vi "Write-Value.vi"(0 "Quick-GUI-Update in":refnum<class "Quick-GUI-Update.lvclass">, 2 "Label":string, 7 "Value In":variant, 11 "error in (no error)":errorcluster) -> (4 "Quick-GUI-Update out":refnum<class "Quick-GUI-Update.lvclass">, 8 "Status":u8[](array[numeric]), 15 "error out":errorcluster)   [LabVIEW 2020, in "Easy GUI Operation.lvlib" / "Quick-GUI-Update.lvclass"]
doc: "<b>Status</b>\n0 ---> Value Not Updated.\n1 ---> Value Updated using <b>\"Set Ctrl Value By Index\"</b> function.\n2 ---> Value Updated using <b>\"Value\"</b> Property."
uses:
  Quick-GUI-Update.lvclass
  Quick-GUI-Update.lvclass/Quick-GUI-Update.ctl
  <vilib>/Utility/Data Type/NI_Data Type.lvlib
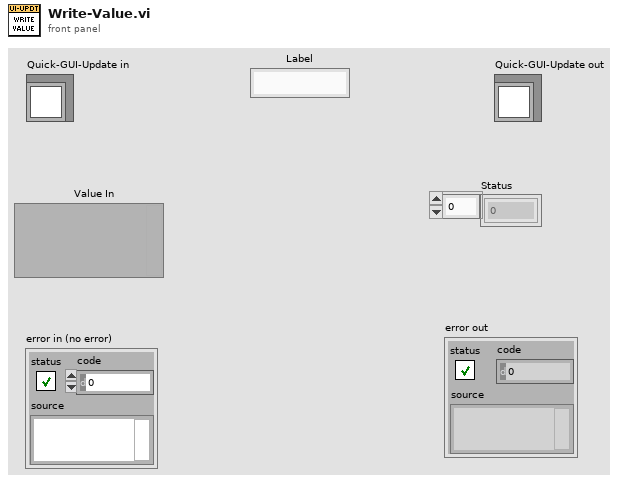
[diagram p1: front panel]
types:
  T1 = map{string, set{cluster{"Ctrl-Ref":refnum<vi>, "Ctrl Index":i32, "Class-Name":string, "Class ID":u32}}}
  T2 = set{cluster{"Ctrl-Ref":refnum<vi>, "Ctrl Index":i32, "Class-Name":string, "Class ID":u32}}
  T3 = typedef "NI_Data Type.lvlib/Data Type.ctl" = enum8{"Invalid Type", "Void", "I8", "I16", "I32", "I64", "U8", "U16", "U32", "U64", "Single Float", "Double Float", "Extended Float", "Single Complex", "Double Complex", "Extended Complex", "Enum U8", "Enum U16", "Enum U32", "Enum U64", "Single Float With Unit", "Double Float With Unit", "Extended Float With Unit", "Single Complex with Unit", "Double Complex with Unit", "Extended Complex with Unit", "Boolean", "String", "Path", "Picture", "Tag", "Array", "Cluster", "Variant", "LV Variant", "Waveform", "Timestamp", "Digital Waveform", "Digital Data", "ExpressData", "Refnum", "External Data", "VI", "Poly VI", "LabVIEW Class Instance", "Fixed Point", "Set Collection", "Map Collection"}
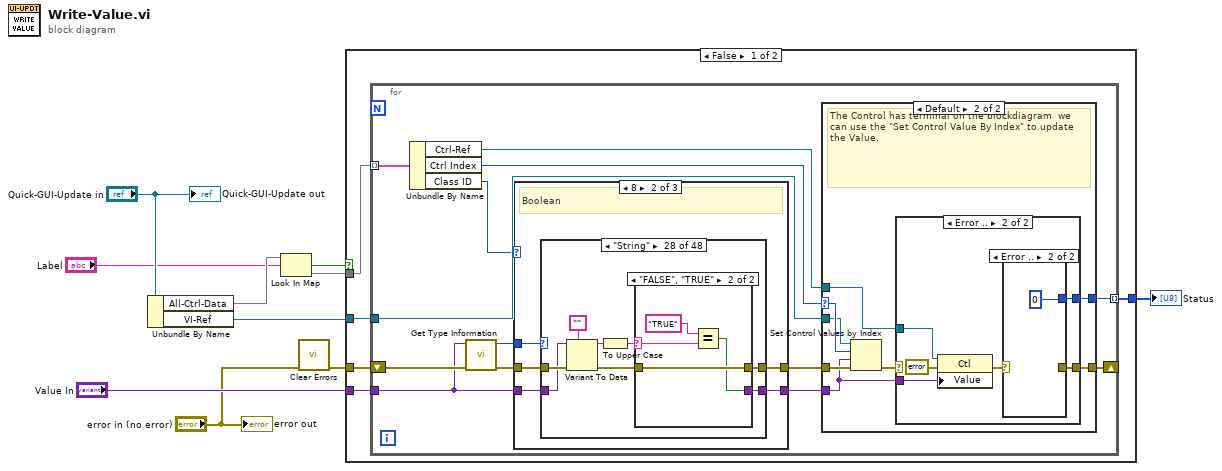
[diagram p0: block diagram]
diagram:
  n1 = Unbundle By Name("Quick-GUI-Update in") -> ("All-Ctrl-Data"=w8:T1, "VI-Ref"=w4:refnum<vi>)
  n2 = Look In Map(map=w8, key="Label") -> (key not found?=w6:bool, value=w5:T2)  [unwired: 1 in]
  n3 = call <vilib>:"Clear Errors.vi"("error in (no error)"="error in (no error)") -> ("error out"=w2:errorcluster)  [unwired: 5 in, 1 out]
  n4 = case shown="False" w6 {
    tunnel: w2 -> [w13 _]
    tunnel: "Value In" -> [w14 _]
    tunnel: w5 -> [w11 _]
    tunnel: w4 -> [w15 _]
    tunnel: [w12 _] -> w3
    frame False {
      n5 = for {
        tunnel: w11 -> [w26] mode=indexing
        tunnel: w15 -> [w24]
        tunnel: w14 -> [w19]
        shift-right: [w25] -> _
        shift-left: w13 -> [w22]
        tunnel: [w23] -> w12 mode=indexing
        n6 = Unbundle By Name(w26) -> ("Ctrl-Ref"=w27:refnum<vi>, "Ctrl Index"=w28:i32, "Class ID"=w21:u32)
        n7 = call <vilib>:"Get Type Information.vi"("error in (no error)"=w22, "variant"=w19) -> ("error out"=w18:errorcluster, "type"=w20:T3)  [unwired: 5 in, 3 out]
        n8 = case shown="8" w21 {
          tunnel: w20 -> [_ w35 w149]
          tunnel: w19 -> [w29 w32 w146]
          tunnel: w18 -> [w30 w34 w148]
          tunnel: [w30 w33 w147] -> w17
          tunnel: [w29 w31 w145] -> w16
          frame Default {
          }
          frame 8 {
            # "Boolean"
            n9 = case shown="\"String\"" w35 {
              tunnel: w34 -> [w37 w39 w41 w43 w45 w47 w49 w51 w53 w55 w57 w59 w61 w63 w65 w67 w69 w71 w73 w75 w77 w79 w81 w83 w85 w87 w89 w97 w106 w108 w110 w112 w114 w116 w118 w120 w122 w124 w126 w128 w130 w132 w134 w136 w138 w140 w142 w144]
              tunnel: [w37 w39 w41 w43 w45 w47 w49 w51 w53 w55 w57 w59 w61 w63 w65 w67 w69 w71 w73 w75 w77 w79 w81 w83 w85 w87 w89 w91 w106 w108 w110 w112 w114 w116 w118 w120 w122 w124 w126 w128 w130 w132 w134 w136 w138 w140 w142 w144] -> w33
              tunnel: w32 -> [w36 w38 w40 w42 w44 w46 w48 w50 w52 w54 w56 w58 w60 w62 w64 w66 w68 w70 w72 w74 w76 w78 w80 w82 w84 w86 w88 w96 w105 w107 w109 w111 w113 w115 w117 w119 w121 w123 w125 w127 w129 w131 w133 w135 w137 w139 w141 w143]
              tunnel: [w36 w38 w40 w42 w44 w46 w48 w50 w52 w54 w56 w58 w60 w62 w64 w66 w68 w70 w72 w74 w76 w78 w80 w82 w84 w86 w88 w92 w105 w107 w109 w111 w113 w115 w117 w119 w121 w123 w125 w127 w129 w131 w133 w135 w137 w139 w141 w143] -> w31
              frame "Invalid Type" {
              }
              frame "Void" {
              }
              frame "I8" {
              }
              frame "I16" {
              }
              frame "I32" {
              }
              frame "I64" {
              }
              frame "U8" {
              }
              frame "U16" {
              }
              frame "U32" {
              }
              frame "U64" {
              }
              frame "Single Float" {
              }
              frame "Double Float" {
              }
              frame "Extended Float" {
              }
              frame "Single Complex" {
              }
              frame "Double Complex" {
              }
              frame "Extended Complex" {
              }
              frame "Enum U8" {
              }
              frame "Enum U16" {
              }
              frame "Enum U32" {
              }
              frame "Enum U64" {
              }
              frame "Single Float With Unit" {
              }
              frame "Double Float With Unit" {
              }
              frame "Extended Float With Unit" {
              }
              frame "Single Complex with Unit" {
              }
              frame "Double Complex with Unit" {
              }
              frame "Extended Complex with Unit" {
              }
              frame "Boolean" {
              }
              frame "String" {
                n10 = Variant To Data(error in=w97, type="" ("Empty String Constant"), Variant=w96) -> (data=w95:string, error out=w93:errorcluster)
                n11 = To Upper Case(1:w95) -> (0:w94:string)
                n12 = case shown="\"FALSE\", \"TRUE\"" w94 {
                  selector: w94 -> [w99 w103]
                  tunnel: w93 -> [w100 w104]
                  tunnel: [w98 w101] -> w92
                  tunnel: [w100 w104] -> w91
                  frame Default {
                    n13 = To Variant(anything=w99) -> (Variant=w98:variant)
                  }
                  frame "FALSE", "TRUE" {
                    n14 = Equal?(x="TRUE", y=w103) -> (x = y?=w101:bool)
                  }
                }
              }
              frame "Path" {
              }
              frame "Picture" {
              }
              frame "Tag" {
              }
              frame "Array" {
              }
              frame "Cluster" {
              }
              frame "Variant" {
              }
              frame "LV Variant" {
              }
              frame "Waveform" {
              }
              frame "Timestamp" {
              }
              frame "Digital Waveform" {
              }
              frame "Digital Data" {
              }
              frame "ExpressData" {
              }
              frame "Refnum" {
              }
              frame "External Data" {
              }
              frame "VI" {
              }
              frame "Poly VI" {
              }
              frame "LabVIEW Class Instance" {
              }
              frame "Fixed Point" {
              }
              frame "Set Collection" {
              }
              frame "Map Collection" {
              }
            }
          }
          frame 27 {
            # "String"
            n15 = case shown="\"Invalid Type\"" w149 {
              tunnel: w148 -> [w151 w153 w155 w157 w159 w161 w163 w165 w167 w169 w171 w173 w175 w177 w179 w181 w183 w185 w187 w189 w191 w193 w195 w197 w199 w201 w208 w210 w212 w214 w216 w218 w220 w222 w224 w226 w228 w230 w232 w234 w236 w238 w240 w242 w244 w246 w248 w250]
              tunnel: [w151 w153 w155 w157 w159 w161 w163 w165 w167 w169 w171 w173 w175 w177 w179 w181 w183 w185 w187 w189 w191 w193 w195 w197 w199 w201 w206 w210 w212 w214 w216 w218 w220 w222 w224 w226 w228 w230 w232 w234 w236 w238 w240 w242 w244 w246 w248 w250] -> w147
              tunnel: w146 -> [w150 w152 w154 w156 w158 w160 w162 w164 w166 w168 w170 w172 w174 w176 w178 w180 w182 w184 w186 w188 w190 w192 w194 w196 w198 w200 w205 w209 w211 w213 w215 w217 w219 w221 w223 w225 w227 w229 w231 w233 w235 w237 w239 w241 w243 w245 w247 w249]
              tunnel: [w150 w152 w154 w156 w158 w160 w162 w164 w166 w168 w170 w172 w174 w176 w178 w180 w182 w184 w186 w188 w190 w192 w194 w196 w198 w200 w202 w209 w211 w213 w215 w217 w219 w221 w223 w225 w227 w229 w231 w233 w235 w237 w239 w241 w243 w245 w247 w249] -> w145
              frame "Invalid Type" {
              }
              frame "Void" {
              }
              frame "I8" {
              }
              frame "I16" {
              }
              frame "I32" {
              }
              frame "I64" {
              }
              frame "U8" {
              }
              frame "U16" {
              }
              frame "U32" {
              }
              frame "U64" {
              }
              frame "Single Float" {
              }
              frame "Double Float" {
              }
              frame "Extended Float" {
              }
              frame "Single Complex" {
              }
              frame "Double Complex" {
              }
              frame "Extended Complex" {
              }
              frame "Enum U8" {
              }
              frame "Enum U16" {
              }
              frame "Enum U32" {
              }
              frame "Enum U64" {
              }
              frame "Single Float With Unit" {
              }
              frame "Double Float With Unit" {
              }
              frame "Extended Float With Unit" {
              }
              frame "Single Complex with Unit" {
              }
              frame "Double Complex with Unit" {
              }
              frame "Extended Complex with Unit" {
              }
              frame "Boolean" {
                n16 = Variant To Data(error in=w208, type=FALSE, Variant=w205) -> (data=w203:bool, error out=w207:errorcluster)
                n17 = Format Into String(error in=w207, w203) -> (resulting string=w202:string, error out=w206:errorcluster)  [unwired: 2 in]
              }
              frame "String" {
              }
              frame "Path" {
              }
              frame "Picture" {
              }
              frame "Tag" {
              }
              frame "Array" {
              }
              frame "Cluster" {
              }
              frame "Variant" {
              }
              frame "LV Variant" {
              }
              frame "Waveform" {
              }
              frame "Timestamp" {
              }
              frame "Digital Waveform" {
              }
              frame "Digital Data" {
              }
              frame "ExpressData" {
              }
              frame "Refnum" {
              }
              frame "External Data" {
              }
              frame "VI" {
              }
              frame "Poly VI" {
              }
              frame "LabVIEW Class Instance" {
              }
              frame "Fixed Point" {
              }
              frame "Set Collection" {
              }
              frame "Map Collection" {
              }
            }
          }
        }
        n18 = case shown="Default" w28 {
          selector: w28 -> [_ w267]
          tunnel: w27 -> [w256 w265]
          tunnel: w16 -> [w255 w262]
          tunnel: w17 -> [w254 w264]
          tunnel: [w251 w263] -> w25
          tunnel: w24 -> [_ w261]
          tunnel: [w253 w260] -> w23
          frame -1 {
            # "The Control has no terminal on the block diagram.  So we can able to use only the \"Value\" property to update the Value."
            n19 = property on="Property Node" class="Ctl"(reference=w256, error in=w254, "Value"=w255) -> (error out=w252:errorcluster)  [unwired: 1 out]
            n20 = case shown="No Error" w252 {
              selector: w252 -> [w257 _]
              tunnel: [u8 2 u8 0] -> w253
              tunnel: [w257 _] -> w251
              frame No Error {
              }
              frame Error {
              }
            }
          }
          frame Default {
            # "The Control has terminal on the blockdiagram  we can use the \"Set Control Value By Index\" to update the Value."
            n21 = Set Control Values by Index(0:w261, 1:w267, 2:w262, 3:w264) -> (11:w266:errorcluster)
            n22 = case shown="Error .." w266 {
              selector: w266 -> [w269 _]
              tunnel: [w269 w270] -> w263
              tunnel: w265 -> [_ w275]
              tunnel: w262 -> [_ w274]
              tunnel: [u8 1 w272] -> w260
              frame No Error {
              }
              frame Error {
                n23 = property on="Property Node" class="Ctl"(reference=w275, error in=errorcluster {"status"=FALSE, "code"=0, "source"=""} ("error in (no error)"), "Value"=w274) -> (error out=w271:errorcluster)  [unwired: 1 out]
                n24 = case shown="Error .." w271 {
                  selector: w271 -> [w276 _]
                  tunnel: [u8 2 u8 0] -> w272
                  tunnel: [w276 _] -> w270
                  frame No Error {
                  }
                  frame Error {
                  }
                }
              }
            }
          }
        }
      }
    }
    frame True {
    }
  }
  "Status" <- w3
  "Quick-GUI-Update out" <- "Quick-GUI-Update in"
  "error out" <- "error in (no error)"
